vi "WaypointAndObstaclesPaint 3.vi"() -> (0 "Sim Course":picture, 3 "?":u8[][](array[numeric]))   [LabVIEW 2014]
panel:
  # "Waypoint and Obstacles Paint 3"
  # "Inputs:"
  # "Outputs:"
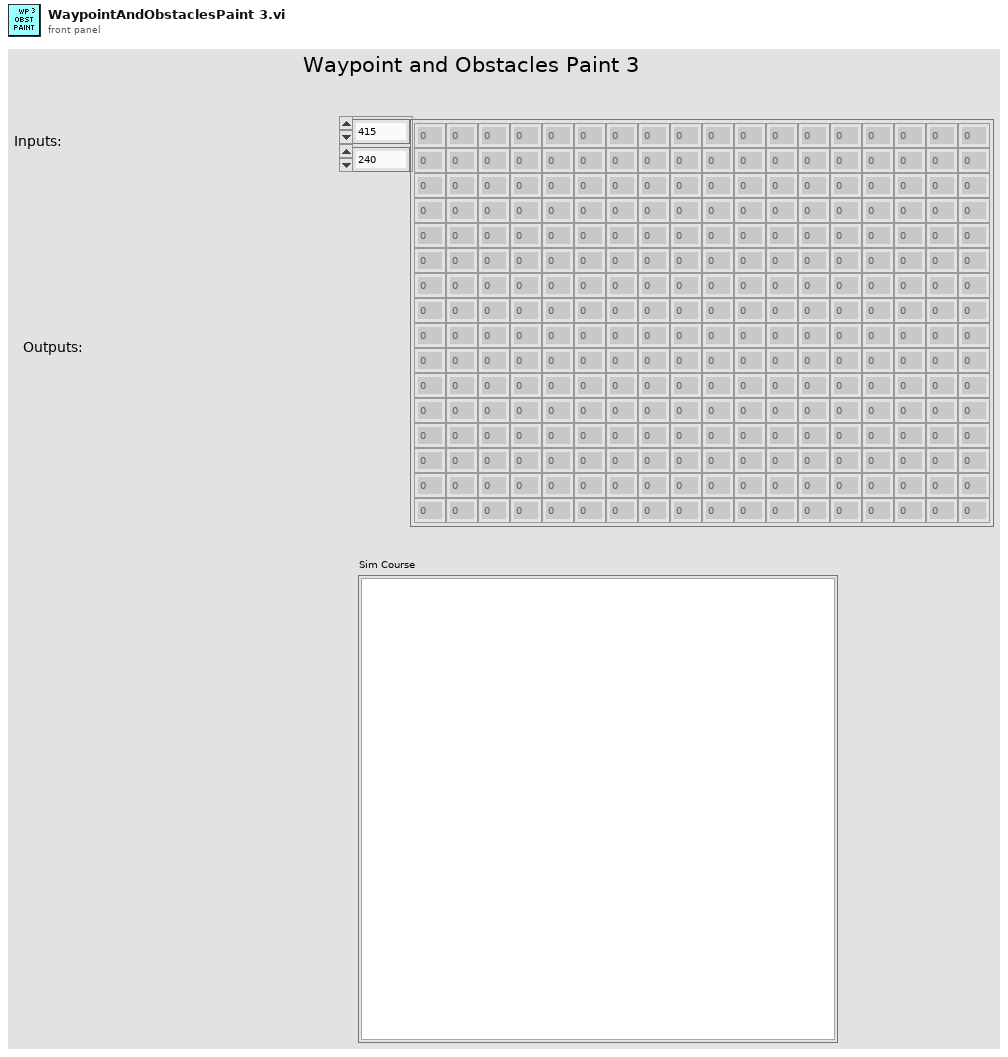
[diagram p1: front panel]
types:
  T1 = typedef "imagedata.ctl" = cluster{"image type":i32, "image depth":i32, "image":u8[], "mask":u8[], "colors":u32[], "Rectangle":cluster{"left":i16, "top":i16, "right":i16, "bottom":i16}}
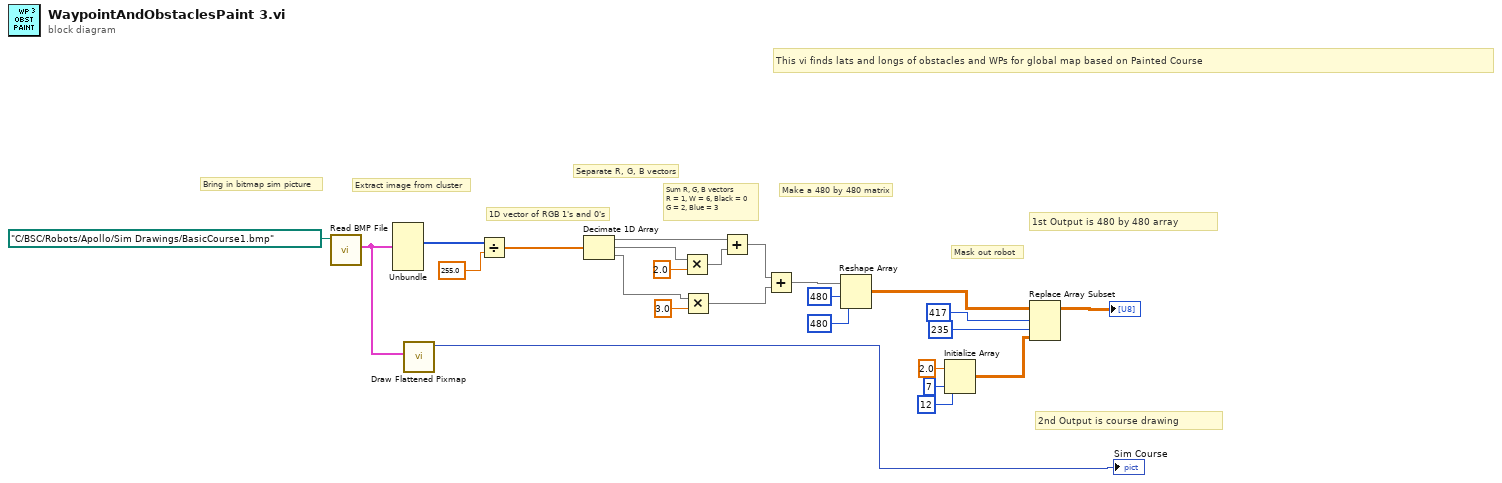
[diagram p0: block diagram]
diagram:
  # "2nd Output is course drawing"
  # "1st Output is 480 by 480 array"
  # "Mask out robot"
  # "Make a 480 by 480 matrix"
  # "Sum R, G, B vectors\nR = 1, W = 6, Black = 0\nG = 2, Blue = 3"
  # "1D vector of RGB 1's and 0's"
  # "This vi finds lats and longs of obstacles and WPs for global map based on Painted Course"
  # "Separate R, G, B vectors"
  # "Extract image from cluster"
  # "Bring in bitmap sim picture"
  n1 = call <vilib>:"Read BMP File.vi"("path to BMP file"=path "C:/BSC/Robots/Apollo/Sim Drawings/BasicCourse1.bmp") -> ("image data"=w2:T1)  [unwired: 8 in, 2 out]
  n2 = Unbundle(w2) -> ("image"=w23:u8[])  [unwired: 5 out]
  n3 = call <vilib>:"Draw Flattened Pixmap.vi"("image data"=w2) -> ("new picture"=→"Sim Course":picture)  [unwired: 8 in]
  n4 = Divide(x=w23, y=255.0) -> (x/y=w22:dbl[])
  n5 = Decimate 1D Array(w22) -> (w14:dbl[], w20:dbl[], w18:dbl[])
  n6 = Multiply(x=w20, y=2.0) -> (x*y=w17:dbl[])
  n7 = Multiply(x=w18, y=3.0) -> (x*y=w15:dbl[])
  n8 = Add(x=w14, y=w17) -> (x+y=w16:dbl[])
  n9 = Add(x=w16, y=w15) -> (x+y=w13:dbl[])
  n10 = Reshape Array(w13, 480 ("dimension size"), 480 ("dimension size")) -> (w5:dbl[][])
  n11 = Initialize Array(2.0 ("element"), 7 ("dimension size"), 12 ("dimension size")) -> (w4:dbl[][])
  n12 = Replace Array Subset(array=w5, new element=w4, index (row)=417, index (col)=235) -> (→"?":dbl[][])
